vi "Read Attributes.vi"(11 "Abstract Message Template in":refnum<class "Publish Analyze Results Msg.lvclass">) -> (2 "Payload":T1, 3 "Abstract Message Template out":refnum<class "Publish Analyze Results Msg.lvclass">)   [LabVIEW 2014, in "Publish Analyze Results Msg.lvclass"]
uses:
  Publish Analyze Results Msg.lvclass
  Analyze/Results and Overlays/Results Base/Analyze Results Base.lvclass
  Analyze/Analyze Parameter/Analyze Parameter Base/Analyze Parameter Base.lvclass
  Publish Analyze Results Msg.lvclass/Publish Analyze Results Msg.ctl
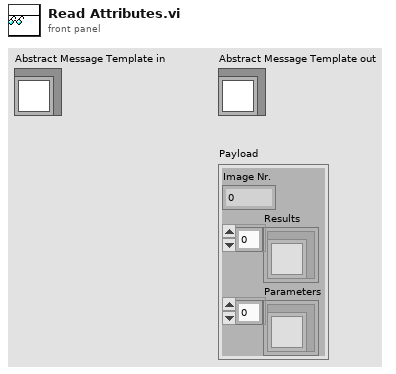
[diagram p1: front panel]
types:
  T1 = cluster{"Image Nr.":i32, "Results":refnum<class "Analyze Results Base.lvclass">[], "Parameters":refnum<class "Analyze Parameter Base.lvclass">[]}
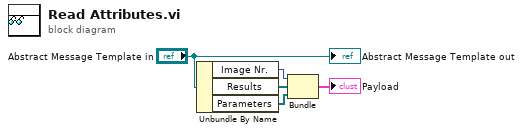
[diagram p0: block diagram]
diagram:
  n1 = Unbundle By Name("Abstract Message Template in") -> ("Image Nr."=w3:i32, "Results"=w4:refnum<class "Analyze Results Base.lvclass">[], "Parameters"=w2:refnum<class "Analyze Parameter Base.lvclass">[])
  n2 = Bundle("Image Nr."=w3, "Results"=w4, "Parameters"=w2) -> (→"Payload":T1)  [unwired: 1 in]
  "Abstract Message Template out" <- "Abstract Message Template in"
